vi "Select INSTR Dialog.vi"() -> (0 "Cancel":bool, 1 "element":string)   [LabVIEW 2015]
doc: "This VI scans for connected USB test and measurement devices. All found devices are shown in a list, where the user can select one of the connected devices. \nOK initialice selected device\nRESCAN look again for connected devices \nCANCEL abort application"
panel:
  in  "Rescan":bool
  in  "Cancel Button":bool
  in  "OK":bool
  in  "Select":i32(listbox) caption="Select Device from List and Press OK"
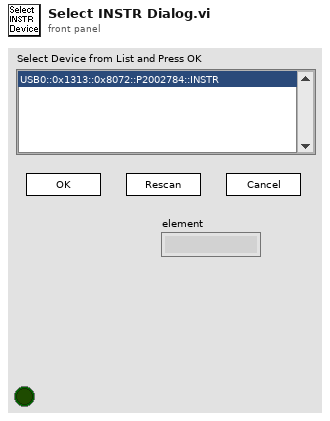
[diagram p1: front panel]
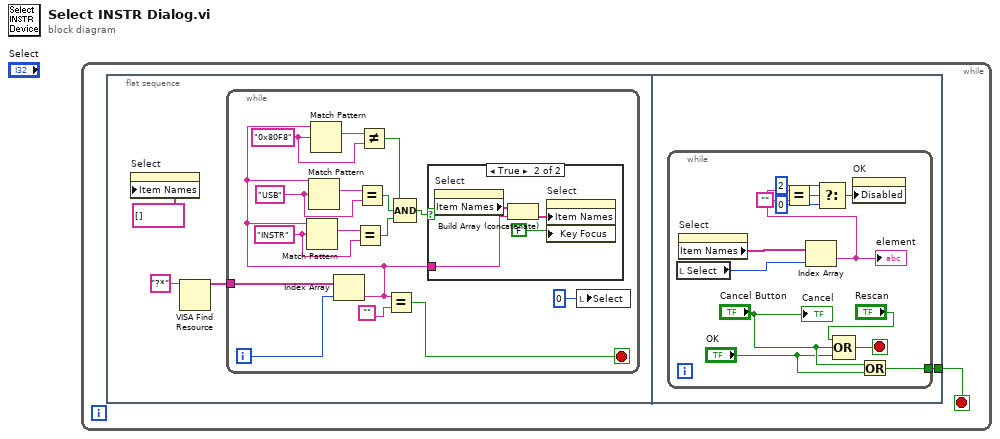
[diagram p0: block diagram]
diagram:
  n1 = while {
    stop <- w1 stop-if-true
    n2 = flat-sequence {
      tunnel: [w25] -> w1
      frame #0 {
        n3 = property on="Select" class="LstBox (strict)"("Item Names"=string[] [] ("Empty")) -> ()  [unwired: 2 in, 2 out]
        n4 = VISA Find Resource(11:"?*" ("expression (\"?*\")")) -> (3:w3:string[])  [unwired: 1 in, 3 out]
        n5 = while {
          tunnel: w3 -> [w12]
          i -> [w11]
          stop <- w10 stop-if-true
          w5 = "0x80F8" ("regular expression")
          w17 = "INSTR" ("regular expression")
          w15 = "USB" ("regular expression")
          n6 = Index Array(array=w12, index=w11) -> (element=w7:string)
          n7 = Match Pattern(string=w7, regular expression=w17) -> (match substring=w16:string)  [unwired: 1 in, 3 out]
          n8 = Match Pattern(string=w7, regular expression=w15) -> (match substring=w14:string)  [unwired: 1 in, 3 out]
          n9 = Match Pattern(string=w7, regular expression=w5) -> (match substring=w8:string)  [unwired: 1 in, 3 out]
          n10 = Equal?(x=w16, y=w17) -> (x = y?=w19:bool)
          n11 = Equal?(x=w14, y=w15) -> (x = y?=w18:bool)
          n12 = Not Equal?(x=w8, y=w5) -> (x != y?=w6:bool)
          n13 = Equal?(x=w7, y="") -> (x = y?=w10:bool)
          n14 = Compound Arithmetic op=AND(w6, w18, w19) -> (w13:bool)
          n15 = case shown="True" w13 {
            tunnel: w7 -> [_ w21]
            frame False {
            }
            frame True {
              n16 = property on="Select" class="LstBox (strict)"() -> ("Item Names"=w23:string[])  [unwired: 2 in, 2 out]
              n17 = Build Array (concatenate)(w23, w21) -> (w22:string[])
              n18 = property on="Select" class="LstBox (strict)"("Item Names"=w22, "Key Focus"=FALSE) -> ()  [unwired: 2 in, 2 out]
            }
          }
          n19 = local write "Select"(0 ("Select Device from List and Press ok")) -> ()
        }
      }
      frame #1 {
        n20 = while {
          tunnel: [w32] -> w25
          stop <- w38 stop-if-true
          n21 = local read "Select"() -> (w37:i32)
          n22 = property on="Select" class="LstBox (strict)"() -> ("Item Names"=w36:string[])  [unwired: 2 in, 2 out]
          n23 = Index Array(array=w36, index=w37) -> (element=w29:string)
          "element" <- w29
          n24 = Equal?(x=w29, y="") -> (x = y?=w30:bool)
          n25 = Select(t=i8 2, s=w30, f=i8 0) -> (s? t:f=w31:i8)
          n26 = Compound Arithmetic op=OR("Rescan", "Cancel Button", "OK") -> (w38:bool)
          n27 = property on="OK" class="Bool"("Disabled"=w31) -> ()  [unwired: 2 in, 2 out]
          n28 = Or(x="Cancel Button", y="OK") -> (x .or. y?=w32:bool)
          "Cancel" <- "Cancel Button"
        }
      }
    }
  }
